vi "UI Communication Loop.vi"(9 "Stream Buffer Size":i32, 10 "Stream Polling Timeout":i32, 11 "Stream Connect Timout":i32) -> ()   [LabVIEW 2018]
uses:
  Global Variables/RT Loop Stop.vi
  Type Defs/UI Communication State.ctl
  Type Defs/Message Cluster.ctl
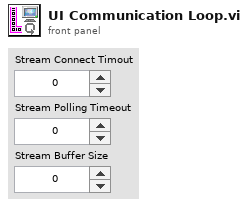
[diagram p1: front panel]
types:
  T1 = typedef "UI Communication State.ctl" = enum16{"Initialize", "Listen for UI Writer", "Receive UI Commands"}
  T2 = typedef "Message Cluster.ctl" = cluster{"Message Data":variant, "Message":string}
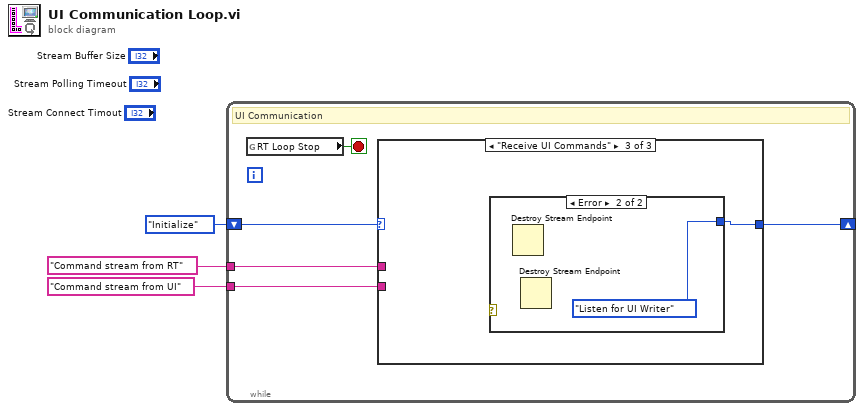
[diagram p0: block diagram]
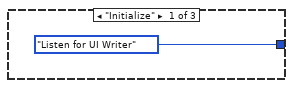
[diagram p2: hidden frame]
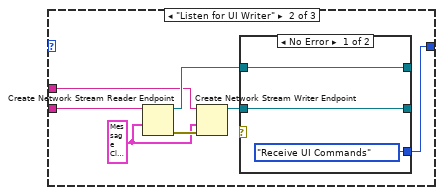
[diagram p3: hidden frame]
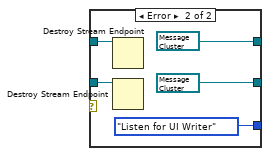
[diagram p4: hidden frame]
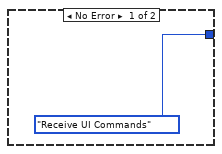
[diagram p5: hidden frame]
diagram:
  n1 = while {
    shift-right: [w6] -> _
    shift-left: UI_Communication_State."Initialize" ("Enum - Menu") -> [w7]
    tunnel: "Command stream from UI" -> [w5]
    tunnel: "Command stream from RT" -> [w4]
    stop <- w8 stop-if-true
    # "UI Communication"
    n2 = global read "RT Loop Stop.vi" "RT Loop Stop"() -> (w8:bool)
    n3 = case shown="\"Receive UI Commands\"" w7 {
      tunnel: [UI_Communication_State."Listen for UI Writer" ("Enum - Menu") w16 w25] -> w6
      tunnel: w5 -> [_ w11 _]
      tunnel: w4 -> [_ w10 _]
      frame "Initialize" {
      }
      frame "Listen for UI Writer" {
        w14 = T2 {"Message Data"=variant, "Message"=""} ("Message Cluster")
        n4 = Create Network Stream Reader Endpoint(9:w14, 11:w11) -> (0:w15:errorcluster, 3:w12:refnum<k21>)  [unwired: 5 in]
        n5 = Create Network Stream Writer Endpoint(8:w15, 9:w14, 11:w10) -> (3:w13:refnum<k21>)  [unwired: 4 in, 1 out]
        n6 = case shown="No Error" {
          selector: _ -> [_ _]
          tunnel: w12 -> [w19 w24]
          tunnel: w13 -> [w18 w23]
          tunnel: [w18 refnum<k21> refnum ("writer endpoint")] -> _
          tunnel: [w19 refnum<k21> refnum ("reader endpoint")] -> _
          tunnel: [UI_Communication_State."Receive UI Commands" ("Enum - Menu") UI_Communication_State."Listen for UI Writer" ("Enum - Menu")] -> w16
          frame No Error {
          }
          frame Error {
            n7 = Destroy Stream Endpoint(11:w24) -> ()  [unwired: 1 in, 1 out]
            n8 = Destroy Stream Endpoint(11:w23) -> ()  [unwired: 1 in, 1 out]
          }
        }
      }
      frame "Receive UI Commands" {
        n9 = case shown="Error" {
          selector: _ -> [_ _]
          tunnel: [UI_Communication_State."Receive UI Commands" ("Enum - Menu") UI_Communication_State."Listen for UI Writer" ("Enum - Menu")] -> w25
          frame No Error {
          }
          frame Error {
            n10 = Destroy Stream Endpoint() -> ()  [unwired: 2 in, 1 out]
            n11 = Destroy Stream Endpoint() -> ()  [unwired: 2 in, 1 out]
          }
        }
      }
    }
  }
